vi "Predict(Dataset)(CuLab).vi"(6 "Dataset":T29={"Dataset_Size"=0, "Dims_In"={"C"=0, "H"=0, "W"=0}, "Labels"=[], "File Paths"=[], "Outputs Ref."=refnum, "Inputs Ref."=variant(refnum<data-value> refnum), "Dims_Out"={"C"=0, "H"=0, "W"=0}}, 8 "error in (no error)":errorcluster, 10 "Feature Scorer Params":T1, 11 "PCore_Instance in":T3={"Dataset_Stats"={"means"={"R"=0.0, "G"=0.0, "B"=0.0}, "vars"={"R"=0.0, "G"=0.0, "B"=0.0}, "DS_Size"=0}, "NN"={"Name"="", "No of Layers"=0, "mBatch"=0, "Layers"=[], "Dimty"=enum."In1D_Out1D", "Dims_In"={"C"=0, "H"=0, "W"=0}, "Dims_Out"={"C"=0, "H"=0, "W"=0}, "Working_Dir"=path "", "Train?"=FALSE, "Train_Params"={"Optimizer"=enum."SGD", "Beta_1"=0.0, "Beta_2"=0.0, "Weight Decay(L1)"=0.0, "Weight Decay(L2)"=0.0, "Data_Sampling"=enum."Random"}, "LR_Update_Policy"={"Policy_Type"=enum."Manual", "LR0"=0.0, "k"=0.0, "WarmUp_Policy"=enum."Step", "WarmUp_Iter"=0, "WarmUp_Ratio"=0.0}, "Session Data"={"Epochs"=0.0, "Tot_Iter"=0, "LR"=0.0, "LR_iter"=0}, "Ground_truth"={"Y"=variant}, "NNg_hdls"={"cudnn"=0, "cublas"=0, "stream"=0, "curand"=0}, "NN_Device"=enum."CPU", "GPU Id"=0, "Labels"=[], "Receptive Field"=[], "Loss_Type"=enum."None", "Loss_Cfg_Prms"=variant, "NNG_WS"={"NNG_WS_Mem"=refnum, "Max_WS_Size"=0}}, "PCore_Device"=enum."CPU", "PatchCore_Init_CFG"={"BackBone"=enum."WRN_50_2_L2L3", "Out_Layers_Names"=[], "Patch_Size"=0}, "Coreset Params"={"Sampling_Ratio"=0.0, "Startd_idx"=0, "Random_Proj?"=FALSE, "Rnd. Proj. Params"={"Proj._Dim."=0, "Epsilon"=0.9, "Seed"=42}}, "MemBank_Data"={"MemBank"=variant, "MemBank Norm"=variant}} {"NN out"."LR_Update_Policy"."WarmUp_Ratio" min=1; "NN out"."LR_Update_Policy"."WarmUp_Iter" min=1; "NN out"."LR_Update_Policy"."LR0" format="%.7f"; "Dataset_Stats"."vars"."R" format="%#_3g"; "Dataset_Stats"."vars"."G" format="%#_3g"; "Dataset_Stats"."vars"."B" format="%#_3g"; "Dataset_Stats"."means"."R" format="%#_3g"; "Dataset_Stats"."means"."G" format="%#_3g"; "Dataset_Stats"."means"."B" format="%#_3g"}) -> (0 "error out":errorcluster, 1 "anomaly maps":refnum<class "T3D_SGL.lvclass">, 2 "pred scores":refnum<class "T1D_SGL.lvclass">, 3 "PCore_Instance out":T3={"Dataset_Stats"={"means"={"R"=0.0, "G"=0.0, "B"=0.0}, "vars"={"R"=0.0, "G"=0.0, "B"=0.0}, "DS_Size"=0}, "NN"={"Name"="", "No of Layers"=0, "mBatch"=0, "Layers"=[], "Dimty"=enum."In1D_Out1D", "Dims_In"={"C"=0, "H"=0, "W"=0}, "Dims_Out"={"C"=0, "H"=0, "W"=0}, "Working_Dir"=path "", "Train?"=FALSE, "Train_Params"={"Optimizer"=enum."SGD", "Beta_1"=0.0, "Beta_2"=0.0, "Weight Decay(L1)"=0.0, "Weight Decay(L2)"=0.0, "Data_Sampling"=enum."Random"}, "LR_Update_Policy"={"Policy_Type"=enum."Manual", "LR0"=0.0, "k"=0.0, "WarmUp_Policy"=enum."Step", "WarmUp_Iter"=0, "WarmUp_Ratio"=0.0}, "Session Data"={"Epochs"=0.0, "Tot_Iter"=0, "LR"=0.0, "LR_iter"=0}, "Ground_truth"={"Y"=variant}, "NNg_hdls"={"cudnn"=0, "cublas"=0, "stream"=0, "curand"=0}, "NN_Device"=enum."CPU", "GPU Id"=0, "Labels"=[], "Receptive Field"=[], "Loss_Type"=enum."None", "Loss_Cfg_Prms"=variant, "NNG_WS"={"NNG_WS_Mem"=refnum, "Max_WS_Size"=0}}, "PCore_Device"=enum."CPU", "PatchCore_Init_CFG"={"BackBone"=enum."WRN_50_2_L2L3", "Out_Layers_Names"=[], "Patch_Size"=0}, "Coreset Params"={"Sampling_Ratio"=0.0, "Startd_idx"=0, "Random_Proj?"=FALSE, "Rnd. Proj. Params"={"Proj._Dim."=0, "Epsilon"=0.9, "Seed"=42}}, "MemBank_Data"={"MemBank"=variant, "MemBank Norm"=variant}} {"NN out"."LR_Update_Policy"."WarmUp_Ratio" min=1; "NN out"."LR_Update_Policy"."WarmUp_Iter" min=1; "NN out"."LR_Update_Policy"."LR0" format="%.7f"; "Dataset_Stats"."vars"."R" format="%#_3g"; "Dataset_Stats"."vars"."G" format="%#_3g"; "Dataset_Stats"."vars"."B" format="%#_3g"; "Dataset_Stats"."means"."R" format="%#_3g"; "Dataset_Stats"."means"."G" format="%#_3g"; "Dataset_Stats"."means"."B" format="%#_3g"}, 5 "dT_Predict(Dataset)(CuLab)":dbl)   [LabVIEW 2020]
doc: "Runs forward propagation over whole dataset of type In3D_Out3D and returns prediction for a pretrained network.\n\n<b>NN in</b> - Network instance input.\n<b>Dataset</b> - A dataset of type In3D_Out3D for which predictions should be generated.\n<b>Predictions</b> - Contains feature maps of the last layer (predictions).\n<b>Predictions</b> - Returns predictions (network outputs) for applied dataset.\n<b>NN out</b> - Network instance output."
uses:
  <vilib>/Ngene/Deep Learning Toolkit/Toolkit/NN_Data/API/DataSet/DataSet_Types/NN_DataSet(In3D_Out3D).ctl
  <vilib>/Ngene/Deep Learning Toolkit/Toolkit/NN_Data/API/NN_Dims(C,H,W).ctl
  <vilib>/Ngene/Deep Learning Toolkit/Toolkit/NN_Data/Controls/DataRef_Types/4D/NN_Data_ref(4D_SGL).ctl
  API/Controls/PatchCore_Instance.ctl
  API/Controls/PatchCore_DS_Stats.ctl
  API/Controls/Image_Stats_RGB.ctl
  <vilib>/Ngene/Deep Learning Toolkit/Toolkit/NN_Network/Controls/NN.ctl
  <vilib>/Ngene/Deep Learning Toolkit/Toolkit/NN_Layers/Controls/NN_Layer_ref.ctl
  <vilib>/Ngene/Deep Learning Toolkit/Toolkit/NN_Layers/Controls/NN_Layer.ctl
  <vilib>/Ngene/Deep Learning Toolkit/Toolkit/NN_Layers/Controls/NN_Layer_Type.ctl
  <vilib>/Ngene/Deep Learning Toolkit/Toolkit/NN_Layers/Controls/NN_Layer_Metrics.ctl
  <vilib>/Ngene/Deep Learning Toolkit/Toolkit/NN_Network/Controls/NN_Device.ctl
  <vilib>/Ngene/Deep Learning Toolkit/Toolkit/NNg/cuda/Controls/nng_cuda_handles.ctl
  <vilib>/Ngene/Deep Learning Toolkit/Toolkit/NN_Layers/Controls/NN_Layer_Dimty.ctl
  <vilib>/Ngene/Deep Learning Toolkit/Toolkit/NN_Layers/Controls/NN_Layer_RF_State.ctl
  <vilib>/Ngene/Deep Learning Toolkit/Toolkit/NN_Data/API/NN_Dims(V,H).ctl
  <vilib>/Ngene/Deep Learning Toolkit/Toolkit/NN_Network/Controls/NN_In_Out_Dim-ty.ctl
  <vilib>/Ngene/Deep Learning Toolkit/Toolkit/NN_Train/Controls/NN_Train_Params.ctl
  <vilib>/Ngene/Deep Learning Toolkit/Toolkit/NN_Train/Controls/NN_Train_Optimizer.ctl
  <vilib>/Ngene/Deep Learning Toolkit/Toolkit/NN_Train/Controls/NN_Train_Data_Sampling.ctl
  <vilib>/Ngene/Deep Learning Toolkit/Toolkit/NN_Train/Controls/NN_LR_Policy_Cfg.ctl
  <vilib>/Ngene/Deep Learning Toolkit/Toolkit/NN_Train/Controls/NN_LR_Policy_Type.ctl
  <vilib>/Ngene/Deep Learning Toolkit/Toolkit/NN_Train/Controls/NN_Train_Session_Data.ctl
  <vilib>/Ngene/Deep Learning Toolkit/Toolkit/NN_Data/Controls/NN_Ground_truth.ctl
  <vilib>/Ngene/Deep Learning Toolkit/Toolkit/NN_Train/Controls/NN_Loss_Type.ctl
  <vilib>/Ngene/Deep Learning Toolkit/Toolkit/NNg/Network/WS/Controls/NNG_WS.ctl
  <vilib>/Ngene/Deep Learning Toolkit/Toolkit/NNg/Network/WS/Controls/NNg_WS_Mem_DVR.ctl
  <vilib>/Ngene/Deep Learning Toolkit/Toolkit/NNg/cuda/Controls/cuda_Mem_desc.ctl
  API/Controls/PCore_Device.ctl
  API/Controls/PatchCore_Init_CFG.ctl
  API/Controls/PatchCore_BackBone_Selector.ctl
  API/Controls/Coreset_Params.ctl
  API/Controls/Random_Projection_Coreset.ctl
  API/Controls/MemBank_and_Norm_Variants.ctl
  API/Controls/Feature_Scorer_Params.ctl
  API/Controls/Gaussian_Blur.ctl
  <vilib>/Ngene/CuLab - GPU Accelerated Toolkit/Toolkit/Low_Level/Tensor_Classes/T_Children/T1D/T1D_Children/T1D_SGL/T1D_SGL.lvclass
  C:/Program Files/National Instruments/LabVIEW 2020/vi.lib/Ngene/CuLab - GPU Accelerated Toolkit/Toolkit/Low_Level/Tensor_Classes/T_Children/T1D/T1D.lvclass
  <vilib>/Ngene/CuLab - GPU Accelerated Toolkit/Toolkit/Low_Level/Tensor_Classes/T_Children/T3D/T3D_Children/T3D_SGL/T3D_SGL.lvclass
  C:/Program Files/National Instruments/LabVIEW 2020/vi.lib/Ngene/CuLab - GPU Accelerated Toolkit/Toolkit/Low_Level/Tensor_Classes/T_Children/T3D/T3D.lvclass
  C:/Program Files/National Instruments/LabVIEW 2020/vi.lib/Ngene/CuLab - GPU Accelerated Toolkit/Toolkit/Low_Level/Tensor_Classes/Tensor.lvclass
  <vilib>/Ngene/CuLab - GPU Accelerated Toolkit/Toolkit/Low_Level/Tensor_Classes/T_Children/T1D/Controls/T1D_Dims.ctl
  <vilib>/Ngene/CuLab - GPU Accelerated Toolkit/Toolkit/Low_Level/Tensor_Classes/T_Children/T3D/Controls/T3D_Dims.ctl
  <vilib>/Ngene/CuLab - GPU Accelerated Toolkit/Toolkit/Low_Level/Tensor_Classes/T_Children/T3D/Controls/T3D_Indices.ctl
  <vilib>/Ngene/CuLab - GPU Accelerated Toolkit/Toolkit/Low_Level/Tensor_Classes/T_Children/T4D/T4D_Children/T4D_SGL/T4D_SGL.lvclass
  <vilib>/Ngene/CuLab - GPU Accelerated Toolkit/Toolkit/API/Array/Array Subset/T1D/CU_Array_Subset_T1D_SGL.vi
  <vilib>/Ngene/CuLab - GPU Accelerated Toolkit/Toolkit/API/Array/Replace Array Subset (API)/CU_Replace_Array_Subset_1D_1D/CU_Replace_Array_Subset_1D_1D_SGL.vi
  <vilib>/Ngene/CuLab - GPU Accelerated Toolkit/Toolkit/API/Array/Array Size/CU_Array_Size_T3D.vi
  <vilib>/Ngene/Deep Learning Toolkit/Toolkit/Deep_Learning_Toolkit_by_Ngene.lvlib
  <vilib>/Ngene/CuLab - GPU Accelerated Toolkit/Toolkit/CuLab.lvlib
  <vilib>/Ngene/CuLab - GPU Accelerated Toolkit/Toolkit/Low_Level/Tensor_Classes/Tensor.lvclass
  C:/Program Files/National Instruments/LabVIEW 2020/vi.lib/Ngene/CuLab - GPU Accelerated Toolkit/Toolkit/Low_Level/Tensor_Classes/T_Children/T3D/T3D_Children/T3D_SGL/T3D_SGL.lvclass
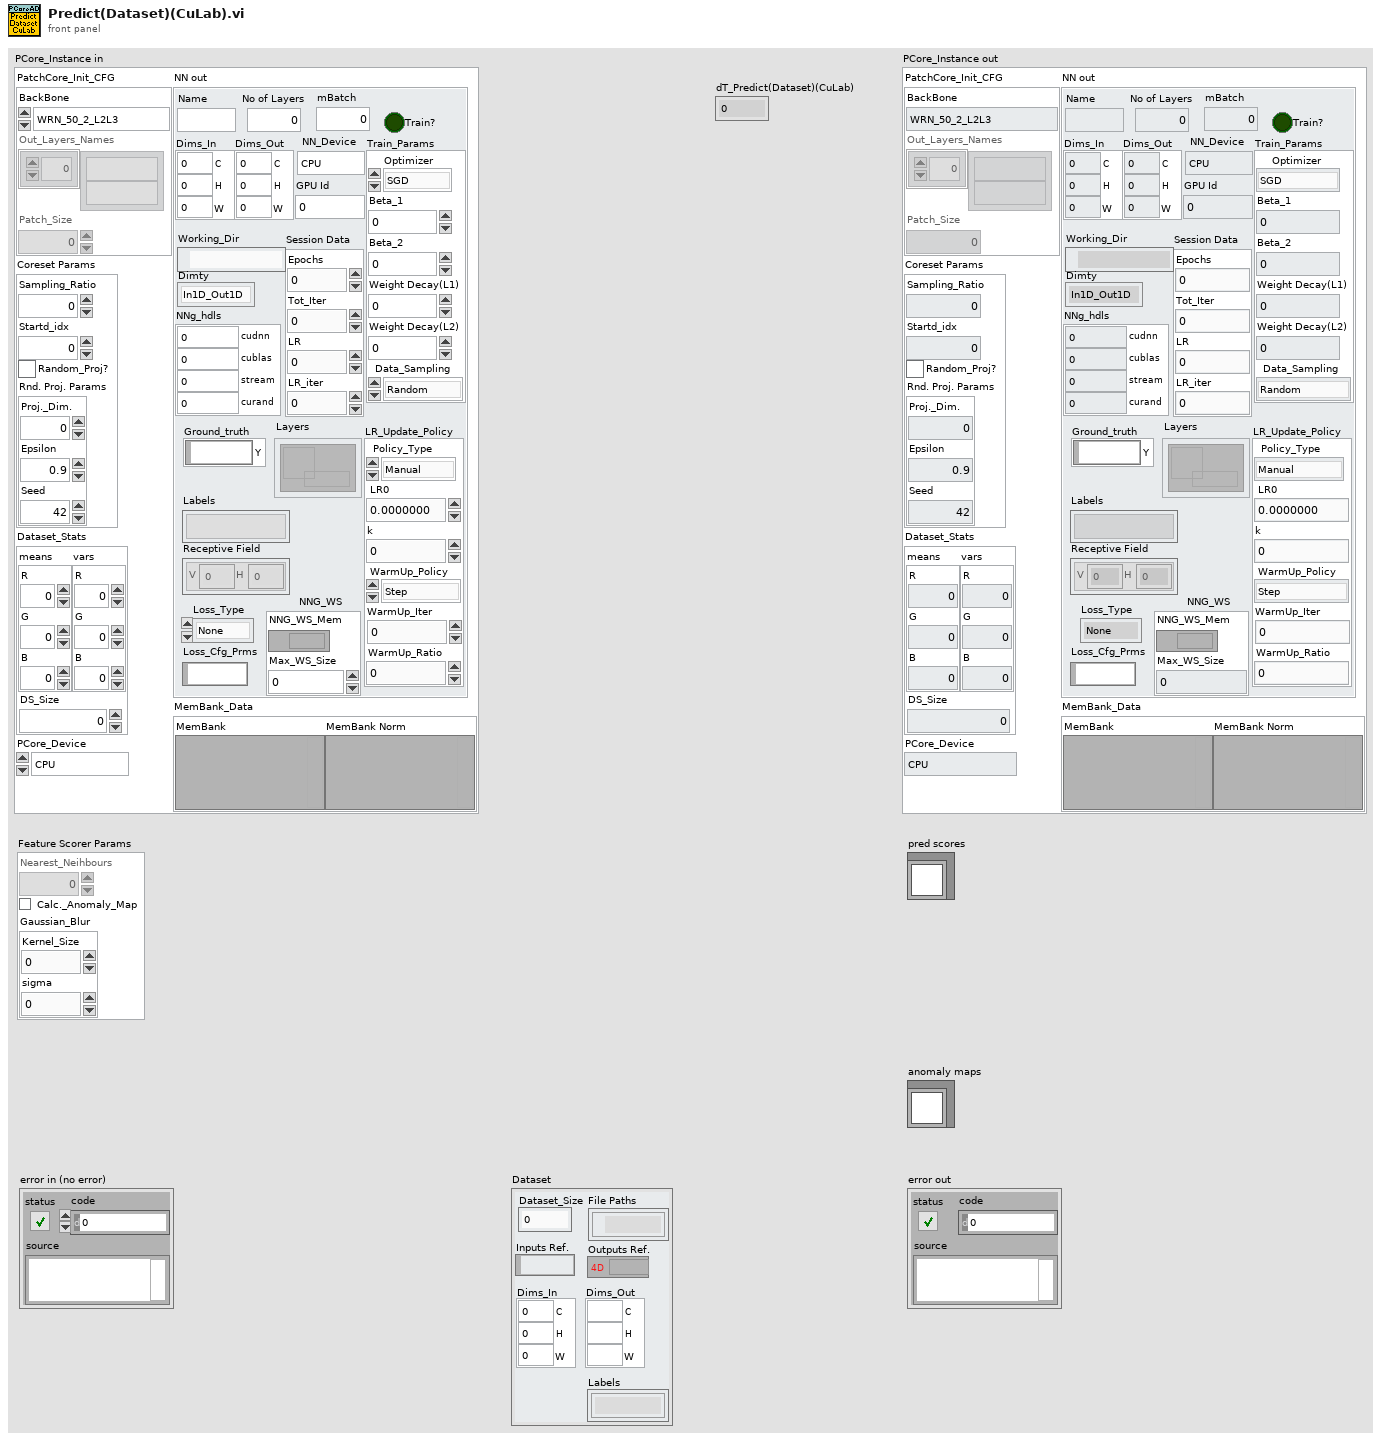
[diagram p1: front panel]
types:
  T1 = typedef "Feature_Scorer_Params.ctl" = cluster{"Nearest_Neihbours":i32, "Calculate Anomaly Map":bool, "Gaussian_Blur":T2}
  T2 = typedef "Gaussian_Blur.ctl" = cluster{"Kernel_Size":i32, "sigma":sgl}
  T3 = typedef "PatchCore_Instance.ctl" = cluster{"Dataset_Stats":T4, "NN":T6, "PCore_Device":T23, "PatchCore_Init_CFG":T24, "Coreset Params":T26, "MemBank_Data":T28}
  T4 = typedef "PatchCore_DS_Stats.ctl" = cluster{"means":T5, "vars":T5, "DS_Size":i32}
  T5 = typedef "Image_Stats_RGB.ctl" = cluster{"R":sgl, "G":sgl, "B":sgl}
  T6 = typedef "Deep_Learning_Toolkit_by_Ngene.lvlib/NN.ctl" = cluster{"Name":string, "No of Layers":i32, "mBatch":i32, "Layers":T7[], "Dimty":T8, "Dims_In":T9, "Dims_Out":T9, "Working_Dir":path, "Train?":bool, "Train_Params":T10, "LR_Update_Policy":T13, "Session Data":T15, "Ground_truth":T16, "NNg_hdls":T17, "NN_Device":T18, "GPU Id":i32, "Labels":string[], "Receptive Field":T19[], "Loss_Type":T20, "Loss_Cfg_Prms":variant, "NNG_WS":T21}
  T7 = typedef "Deep_Learning_Toolkit_by_Ngene.lvlib/NN_Layer_ref.ctl" = refnum<data-value>
  T8 = typedef "Deep_Learning_Toolkit_by_Ngene.lvlib/NN_In_Out_Dim-ty.ctl" = enum8{"In1D_Out1D", "In3D_Out1D", "In3D_Out3D", "In3D_OutBBox"}
  T9 = typedef "Deep_Learning_Toolkit_by_Ngene.lvlib/NN_Dims(C,H,W).ctl" = cluster{"C":i32, "H":i32, "W":i32}
  T10 = typedef "Deep_Learning_Toolkit_by_Ngene.lvlib/NN_Train_Params.ctl" = cluster{"Optimizer":T11, "Beta_1":sgl, "Beta_2":sgl, "Weight Decay(L1)":sgl, "Weight Decay(L2)":sgl, "Data_Sampling":T12}
  T11 = typedef "Deep_Learning_Toolkit_by_Ngene.lvlib/NN_Train_Optimizer.ctl" = enum16{"SGD", "Adam", "Adagrad", "Adadelta", "RMSProp", "Nesterov"}
  T12 = typedef "Deep_Learning_Toolkit_by_Ngene.lvlib/NN_Train_Data_Sampling.ctl" = enum16{"Random", "Sequential"}
  T13 = typedef "Deep_Learning_Toolkit_by_Ngene.lvlib/NN_LR_Policy_Cfg.ctl" = cluster{"Policy_Type":T14, "LR0":dbl, "k":sgl, "WarmUp_Policy":enum16{"Step", "Ramp"}, "WarmUp_Iter":i32, "WarmUp_Ratio":sgl}
  T14 = typedef "Deep_Learning_Toolkit_by_Ngene.lvlib/NN_LR_Policy_Type.ctl" = enum16{"Manual", "Step", "Exp", "1/t"}
  T15 = typedef "Deep_Learning_Toolkit_by_Ngene.lvlib/NN_Train_Session_Data.ctl" = cluster{"Epochs":sgl, "Tot_Iter":i32, "LR":sgl, "LR_iter":i32}
  T16 = typedef "Deep_Learning_Toolkit_by_Ngene.lvlib/NN_Ground_truth.ctl" = cluster{"Y":variant}
  T17 = typedef "Deep_Learning_Toolkit_by_Ngene.lvlib/nng_cuda_handles.ctl" = cluster{"cudnn":u64, "cublas":u64, "stream":u64, "curand":u64}
  T18 = typedef "Deep_Learning_Toolkit_by_Ngene.lvlib/NN_Device.ctl" = enum16{"CPU", "GPU"}
  T19 = typedef "Deep_Learning_Toolkit_by_Ngene.lvlib/NN_Dims(V,H).ctl" = cluster{"V":i32, "H":i32}
  T20 = typedef "Deep_Learning_Toolkit_by_Ngene.lvlib/NN_Loss_Type.ctl" = enum16{"None", "MSE", "CrossEntropy", "YOLO_v2", "YOLO_v4"}
  T21 = typedef "Deep_Learning_Toolkit_by_Ngene.lvlib/NNG_WS.ctl" = cluster{"NNG_WS_Mem":T22, "Max_WS_Size":i64}
  T22 = typedef "Deep_Learning_Toolkit_by_Ngene.lvlib/NNg_WS_Mem_DVR.ctl" = refnum<data-value>
  T23 = typedef "PCore_Device.ctl" = enum16{"CPU", "GPU(CuLab)"}
  T24 = typedef "PatchCore_Init_CFG.ctl" = cluster{"BackBone":T25, "Out_Layers_Names":string[], "Patch_Size":u32}
  T25 = typedef "PatchCore_BackBone_Selector.ctl" = enum16{"WRN_50_2_L2L3"}
  T26 = typedef "Coreset_Params.ctl" = cluster{"Sampling_Ratio":sgl, "Startd_idx":i32, "Random_Proj?":bool, "Rnd. Proj. Params":T27}
  T27 = typedef "Random_Projection_Coreset.ctl" = cluster{"Proj._Dim.":i32, "Epsilon":sgl, "Seed":i32}
  T28 = typedef "MemBank_and_Norm_Variants.ctl" = cluster{"MemBank":variant, "MemBank Norm":variant}
  T29 = typedef "Deep_Learning_Toolkit_by_Ngene.lvlib/NN_DataSet(In3D_Out3D).ctl" = cluster{"Dataset_Size":i32, "Dims_In":T9, "Labels":string[], "File Paths":path[], "Outputs Ref.":T30, "Inputs Ref.":variant, "Dims_Out":T9}
  T30 = typedef "Deep_Learning_Toolkit_by_Ngene.lvlib/NN_Data_ref(4D_SGL).ctl" = refnum<data-value>
  T31 = typedef "CuLab.lvlib/T1D_Dims.ctl" = cluster{"W":i32}
  T32 = typedef "CuLab.lvlib/T3D_Indices.ctl" = cluster{"k ":i32, "i":i32, "j":i32}
  T33 = typedef "CuLab.lvlib/T3D_Dims.ctl" = cluster{"C ":i32, "H":i32, "W":i32}
  T34 = typedef "Deep_Learning_Toolkit_by_Ngene.lvlib/NN_Layer.ctl" = cluster{"Name":string, "Layer_Data":variant, "Layer_Type":T35, "Dims_In":T9, "Layers_In":variant, "Dims_Out":T9, "Layers_Out":variant, "Metrics":T36, "GPU_Data":variant, "mBatch":i32, "NN_Device":T18, "NNg_hdls":T17, "Train?":bool, "Dimty":T37, "RecptField":T38}
  T35 = typedef "Deep_Learning_Toolkit_by_Ngene.lvlib/NN_Layer_Type.ctl" = enum16{"Input1D", "Input3D", "Conv1D", "Conv2D", "Conv2D_Adv", "MaxPool", "AvgPool", "UpSample", "DropOut3D", "ShortCut", "Concat", "SoftMax3D", "FC", "DropOut", "Softmax", "Flatten", "YOLO_v2", "YOLO_v4", "Activation", "BatchNormalization", "Unsupported"}
  T36 = typedef "Deep_Learning_Toolkit_by_Ngene.lvlib/NN_Layer_Metrics.ctl" = cluster{"Data":dbl, "Params":dbl, "Ops":dbl}
  T37 = typedef "Deep_Learning_Toolkit_by_Ngene.lvlib/NN_Layer_Dimty.ctl" = enum16{"1D", "3D"}
  T38 = typedef "Deep_Learning_Toolkit_by_Ngene.lvlib/NN_Layer_RF_State.ctl" = cluster{"Dims":T19, "J":T19}
  T39 = typedef "CuLab.lvlib/cudart_DataType.ctl" = enum16{"I8", "U8", "I16", "U16", "I32", "U32", "I64", "U64", "SGL", "DBL", "CSG", "CDB"}
  T40 = typedef "CuLab.lvlib/cudart_Mem_desc.ctl" = cluster{"Ref*":u64, "Size(B)":u64}
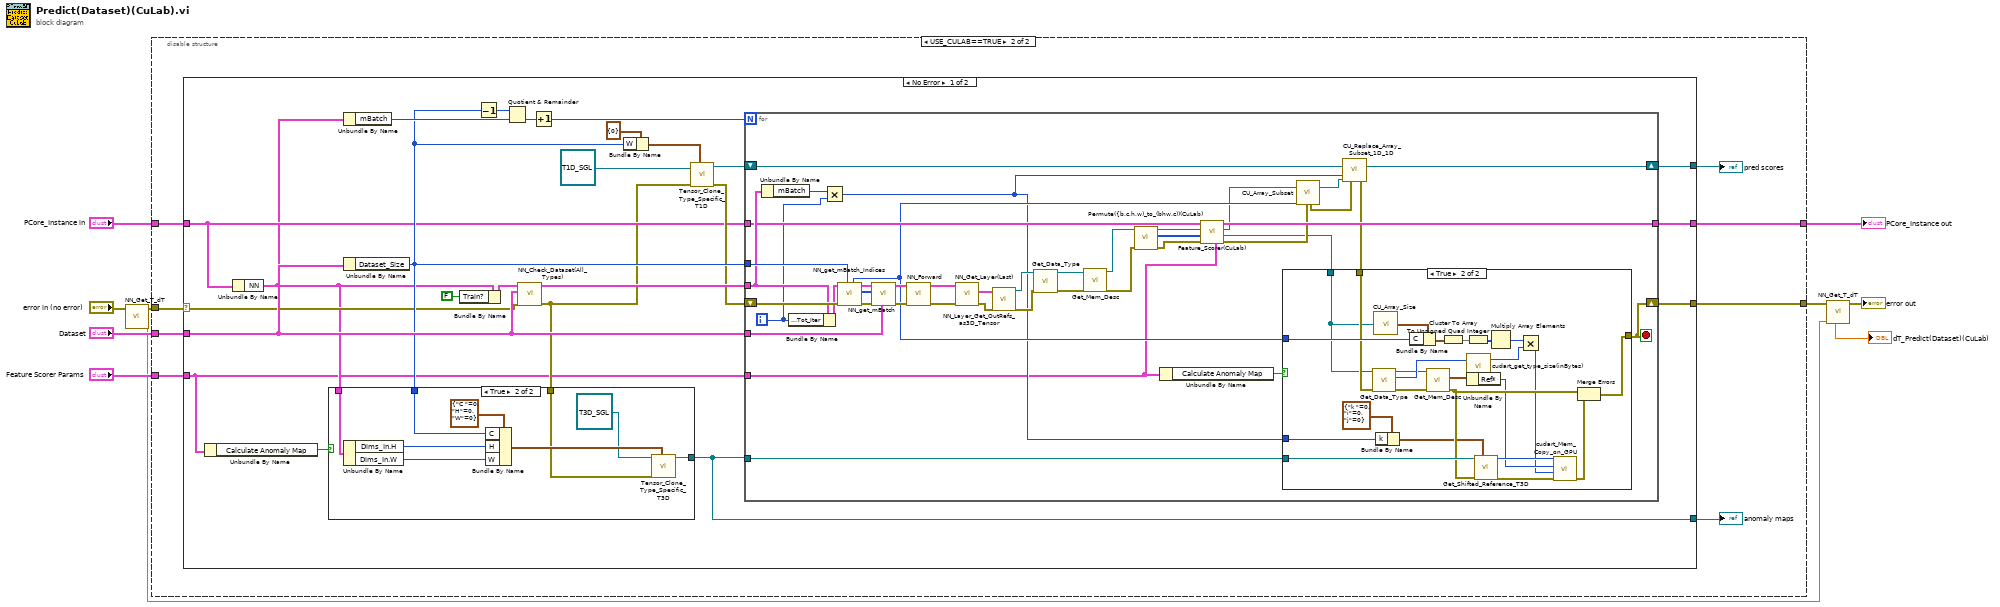
[diagram p0: block diagram]
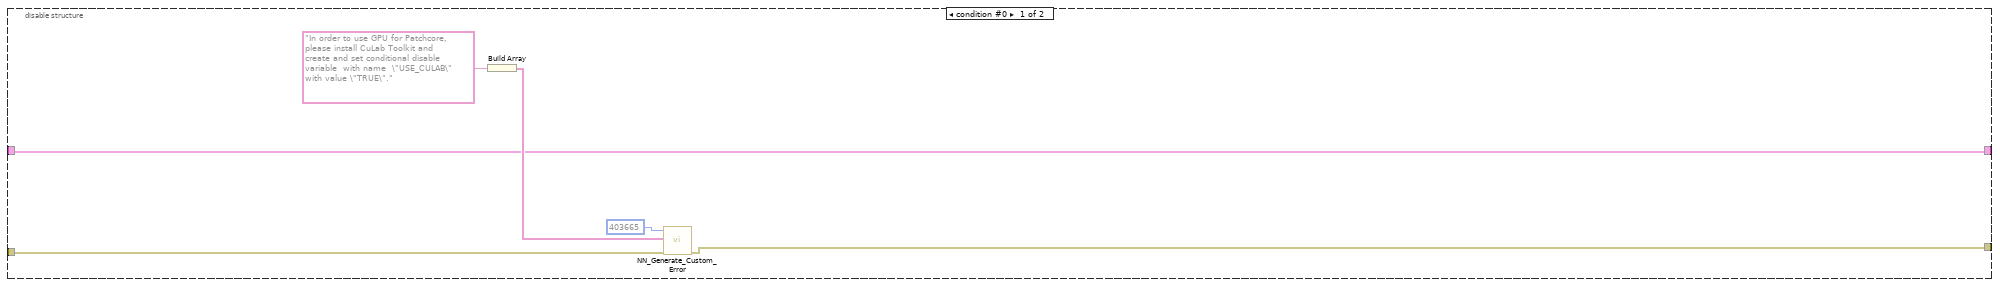
[diagram p2: hidden frame]
diagram:
  n1 = call <vilib>:"NN_Get_T_dT.vi"("error in (no error)"="error in (no error)") -> ("T_out"=w2:dbl, "error out"=w4:errorcluster)  [unwired: 6 in, 1 out]
  n2 = disable-structure shown="USE_CULAB==TRUE" {
    disable-tunnel: "Dataset" -> [_ w24]
    disable-tunnel: w4 -> [w13 w23]
    disable-tunnel: [w12 w22] -> w8
    disable-tunnel: "PCore_Instance in" -> [w11 w21]
    disable-tunnel: "Feature Scorer Params" -> [_ w20]
    disable-tunnel: [w11 w19] -> w6
    frame condition #0 {
      n3 = Build Array("In order to use GPU for Patchcore, please install CuLab Toolkit and create and set conditional disable variable  with name  \"USE_CULAB\" with value \"TRUE\"." ("Message")) -> (w15:string[])
      n4 = call <vilib>:"NN_Generate_Custom_Error.vi"("error in (no error)"=w13, "Message"=w15, "Error_code"=403665) -> ("error out"=w12:errorcluster)  [unwired: 8 in]
    }
    frame condition #1 (active) {
      n5 = case shown="No Error" w23 {
        selector: w23 -> [w33 w125]
        tunnel: w24 -> [w41 _]
        tunnel: [w35 w125] -> w22
        tunnel: w21 -> [w30 w124]
        tunnel: w20 -> [w26 _]
        tunnel: [w36 w124] -> w19
        tunnel: [w27 _] -> w18
        tunnel: [w31 _] -> w17
        frame No Error {
          n6 = Unbundle By Name(w26) -> ("Calculate Anomaly Map"=w25:bool)
          n7 = Unbundle By Name(w30) -> ("NN"=w29:T6)
          n8 = Unbundle By Name(w29) -> ("mBatch"=w43:i32)
          n9 = Unbundle By Name(w41) -> ("Dataset_Size"=w34:i32)
          n10 = Bundle By Name(cluster=w29, "Train?"=FALSE) -> (w48:T6)
          n11 = Decrement(x=w34) -> (x-1=w46:i32)
          n12 = Quotient & Remainder(x=w46, y=w43) -> (floor(x/y)=w45:i32)  [unwired: 1 out]
          n13 = call <vilib>:"NN_Check_Dataset(All_Types).vi"("error in (no error)"=w33, "Train DataSet"=w41, "NN in"=w48) -> ("error out"=w28:errorcluster, "NN out"=w42:T6)  [unwired: 5 in, 2 out]
          n14 = case shown="True" w25 {
            tunnel: w34 -> [_ w122]
            tunnel: w29 -> [_ w119]
            tunnel: w28 -> [_ w117]
            tunnel: [_ w115] -> w27
            frame False {
            }
            frame True {
              n15 = Unbundle By Name(w119) -> ("Dims_In.H"=w121:i32, "Dims_In.W"=w120:i32)
              n16 = Bundle By Name(cluster=T33 {"C "=0, "H"=0, "W"=0} ("Dest Dims"), "C"=w122, "H"=w121, "W"=w120) -> (w118:T33)
              n17 = call <vilib>:"Tensor_Clone_Type_Specific_T3D.vi"("Dest_Tensor_Dims"=w118, "error in (no error)"=w117, "Dest_Tensor"=refnum<class "T3D_SGL.lvclass"> refnum ("Dest out")) -> ("Dest_Tensor out"=w115:refnum<class "T3D_SGL.lvclass">)  [unwired: 7 in, 1 out]
            }
          }
          n18 = Increment(x=w45) -> (x+1=w44:i32)
          n19 = Bundle By Name(cluster=T31 {"W"=0} ("Dest_Tensor_Dims"), "W"=w34) -> (w39:T31)
          n20 = call <vilib>:"Tensor_Clone_Type_Specific_T1D.vi"("Dest_Tensor_Dims"=w39, "error in (no error)"=w28, "Dest_Tensor"=refnum<class "T1D_SGL.lvclass"> refnum ("pred score")) -> ("error out"=w32:errorcluster, "Dest_Tensor out"=w37:refnum<class "T1D_SGL.lvclass">)  [unwired: 7 in]
          n21 = for {
            N: w44 -> [_]
            shift-right: [w52] -> w35
            shift-left: w32 -> [w84]
            tunnel: w41 -> [w72]
            tunnel: w42 -> [w75]
            tunnel: w34 -> [w81]
            tunnel: w30 -> [w68]
            tunnel: w26 -> [w50]
            tunnel: [w64] -> w36
            shift-right: [w61] -> w31
            shift-left: w37 -> [w63]
            tunnel: w27 -> [w54]
            i -> [w62]
            stop <- w52 stop-if-true
            n22 = Unbundle By Name(w75) -> ("mBatch"=w74:i32)
            n23 = Bundle By Name(cluster=w75, "Session Data.Tot_Iter"=w62) -> (w82:T6)
            n24 = Multiply(x=w74, y=w62) -> (x*y=w53:i32)
            n25 = call <vilib>:"NN_get_mBatch_Indices.vi"("Dataset_Size"=w81, "error in (no error)"=w84, "NN in"=w82) -> ("error out"=w83:errorcluster, "Indices"=w80:i32[], "NN Out"=w85:T6, "Actual mBatch Size"=w58:i32)  [unwired: 5 in]
            n26 = call <vilib>:"NN_get_mBatch.vi"("DataSet"=w72, "error in (no error)"=w83, "Indices"=w80, "NN in"=w85) -> ("error out"=w87:errorcluster, "NN Out"=w88:T6)  [unwired: 5 in, 1 out]
            n27 = call <vilib>:"NN_Forward.vi"("error in (no error)"=w87, "NN in"=w88) -> ("error out"=w86:errorcluster, "NN out"=w89:T6)  [unwired: 6 in, 2 out]
            n28 = call <vilib>:"NN_Get_Layer(Last).vi"("error in (no error)"=w86, "NN in"=w89) -> ("error out"=w78:errorcluster, "Last_Layer"=w79:T34)  [unwired: 6 in, 2 out]
            n29 = call "NN_Layer_Get_OutRefs_as3D_Tensor.vi"("error in (no error)"=w78, "Layer"=w79) -> ("error out"=w71:errorcluster, "Out"=w76:refnum<class "T4D_SGL.lvclass">)  [unwired: 7 in, 1 out]
            n30 = call-dynamic "Get_Data_Type.vi"("error in (no error)"=w71, "T4D_SGL in"=w76) -> ("error out"=w73:errorcluster, "T4D_SGL out"=w77:refnum<class "T4D_SGL.lvclass">)  [unwired: 7 in, 1 out]
            n31 = call <vilib>:"Get_Mem_Desc.vi"("error in (no error)"=w73, "Tensor in"=w77) -> ("error out"=w66:errorcluster, "Tensor out"=w70:refnum<class "T4D_SGL.lvclass">)  [unwired: 5 in, 3 out]
            n32 = call "Permute({b,c,h,w)_to_(bhw,c))(CuLab).vi"("error in"=w66, "Features (bs, (c1+c2+...+cN), h, w)"=w70) -> ("error out"=w67:errorcluster, "Orig dims (bs, h, w, (c1+c2+...+cN))"=w65:i32[], "Features reshaped ((bs  x h x w),  c1+c1+..+ cN )"=w69:refnum<class "T2D_SGL.lvclass">)  [unwired: 6 in, 1 out]
            n33 = Unbundle By Name(w50) -> ("Calculate Anomaly Map"=w49:bool)
            n34 = call "Feature_Scorer(CuLab).vi"("Feature Scorer Params"=w50, "error in"=w67, "bs, h, w, c1+..cN"=w65, "embedding"=w69, "PCore_Instance"=w68) -> ("error out"=w60:errorcluster, "anomaly map"=w51:refnum<class "T3D_SGL.lvclass">, "pred score"=w57:refnum<class "T1D_SGL.lvclass">, "PCore_Instance out"=w64:T3)  [unwired: 2 in, 1 out]
            n35 = call-poly <vilib>:"CU_Array_Subset.vi"("Tensor in"=w57, "Length"=w58, "error in (no error)"=w60) -> ("error out"=w59:errorcluster, "Dest out"=w56:refnum<class "T1D_SGL.lvclass">)  [unwired: 15 in]
            n36 = call-poly <vilib>:"CU_Replace_Array_Subset_1D_1D.vi"("Tensor in"=w63, "index"=w53, "Sub Tensor"=w56, "error in (no error)"=w59) -> ("Tensor Out"=w61:refnum<class "T1D_SGL.lvclass">, "error out"=w55:errorcluster)  [unwired: 10 in]
            n37 = case shown="True" w49 {
              tunnel: w58 -> [_ w105]
              tunnel: w55 -> [w90 w104]
              tunnel: w54 -> [_ w103]
              tunnel: w53 -> [_ w99]
              tunnel: [w90 w94] -> w52
              tunnel: w51 -> [_ w91]
              frame False {
              }
              frame True {
                n38 = call-dynamic "Get_Data_Type.vi"("error in (no error)"=w104, "T3D_SGL in"=w91) -> ("error out"=w108:errorcluster, "DataType"=w110:T39, "T3D_SGL out"=w109:refnum<class "T3D_SGL.lvclass">)  [unwired: 7 in]
                n39 = call-poly <vilib>:"CU_Array_Size.vi"("Tensor"=w91) -> ("T3D_Dims"=w106:T33)  [unwired: 14 in]
                n40 = Bundle By Name(cluster=T32 {"k "=0, "i"=0, "j"=0} ("Indices"), "k"=w99) -> (w100:T32)
                n41 = Bundle By Name(cluster=w106, "C"=w105) -> (w114:T33)
                n42 = call <vilib>:"Get_Mem_Desc.vi"("error in (no error)"=w108, "Tensor in"=w109) -> ("error out"=w102:errorcluster, "Mem_Desc"=w107:T40)  [unwired: 5 in, 3 out]
                n43 = Cluster To Array(cluster=w114) -> (array=w111:i32[])
                n44 = To Unsigned Quad Integer(1:w111) -> (0:w112:u64[])
                n45 = Unbundle By Name(w107) -> ("Ref*"=w96:u64)
                n46 = call <vilib>:"cudart_get_type_size(inBytes).vi"("DataType_t"=w110) -> ("Size in Bytes"=w92:u64)  [unwired: 2 in]
                n47 = call <vilib>:"Get_Shifted_Reference_T3D.vi"("Tensor"=w103, "Indices"=w100, "error in (no error)"=w102) -> ("Ref* out"=w98:u64, "error out"=w97:errorcluster)  [unwired: 11 in]
                n48 = Multiply Array Elements(1:w112) -> (0:w113:u64)
                n49 = Multiply(x=w113, y=w92) -> (x*y=w95:u64)
                n50 = call <vilib>:"cudart_Mem_Copy_on_GPU.vi"("error in (no error)"=w97, "size"=w95, "src"=w96, "dest"=w98) -> ("error out"=w93:errorcluster)  [unwired: 6 in, 1 out]
                n51 = Merge Errors(w102, w93) -> (w94:errorcluster)
              }
            }
          }
        }
        frame Error {
        }
      }
      "pred scores" <- w17
      "anomaly maps" <- w18
    }
  }
  "PCore_Instance out" <- w6
  n52 = call <vilib>:"NN_Get_T_dT.vi"("T_in"=w2, "error in (no error)"=w8) -> ("error out"=→"error out":errorcluster, "dT"=→"dT_Predict(Dataset)(CuLab)":dbl)  [unwired: 5 in, 1 out]
